vi "CRYTree Refresh Configure Info.vi"(0 "sOption":string, 5 "Step":T1 {"Repeat State Array"."Start" format="%#_5g"; "Y dB ref" format="%.1f"; "Y data" items=["dB", "Lin"]; "Start" format="%#_5g"}, 7 "Item Indent":i32, 9 "Child3":string, 11 "Child4":string, 12 "SpaceStr":string, 13 "Child5":string) -> (4 "Tree Items":T2(array[cluster]))   [LabVIEW 2013]
uses:
  CRYSystem/Typedef Control/CRYStep.ctl
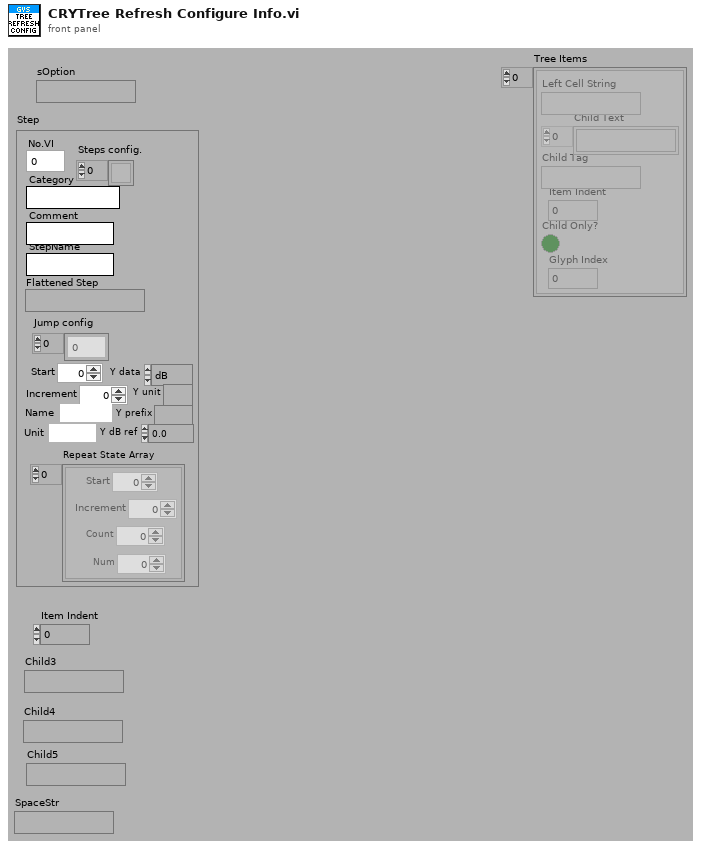
[diagram p1: front panel]
types:
  T1 = typedef "CRYStep.ctl" = cluster{"No.VI":i32, "Category":string, "StepName":string, "Seq setup flattened":string, "Comment":string, "Steps config.":bool[], "Jump config":i32[], "Start":dbl, "Increment":dbl, "Name":string, "Unit":string, "Y data":u16, "Y prefix":string, "Y dB ref":dbl, "Y unit":string, "Repeat State Array":cluster{"Start":dbl, "Increment":dbl, "Count":i32, "Num":i32}[]}
  T2 = cluster{"Left Cell String":string, "Child Text":string[], "Child Tag":string, "Item Indent":i32, "Child Only?":bool, "Glyph Index":i32}[]
  T3 = cluster{"Left Cell String":string, "Child Text":string[], "Child Tag":string, "Item Indent":i32, "Child Only?":bool, "Glyph Index":i32}
  T4 = typedef "CRYStart Cluster.ctl" = cluster{"SequenceName":string, "Preload Stimulus":bool, "CloseOpenedDisplay":bool, "ClearMeasuredData":bool, "UpdateDisplayDuringRun":bool, "DisplayForConfirmation":bool, "HaltOnFail":bool, "UseSameHardware":bool, "UseSameCalibration":bool}
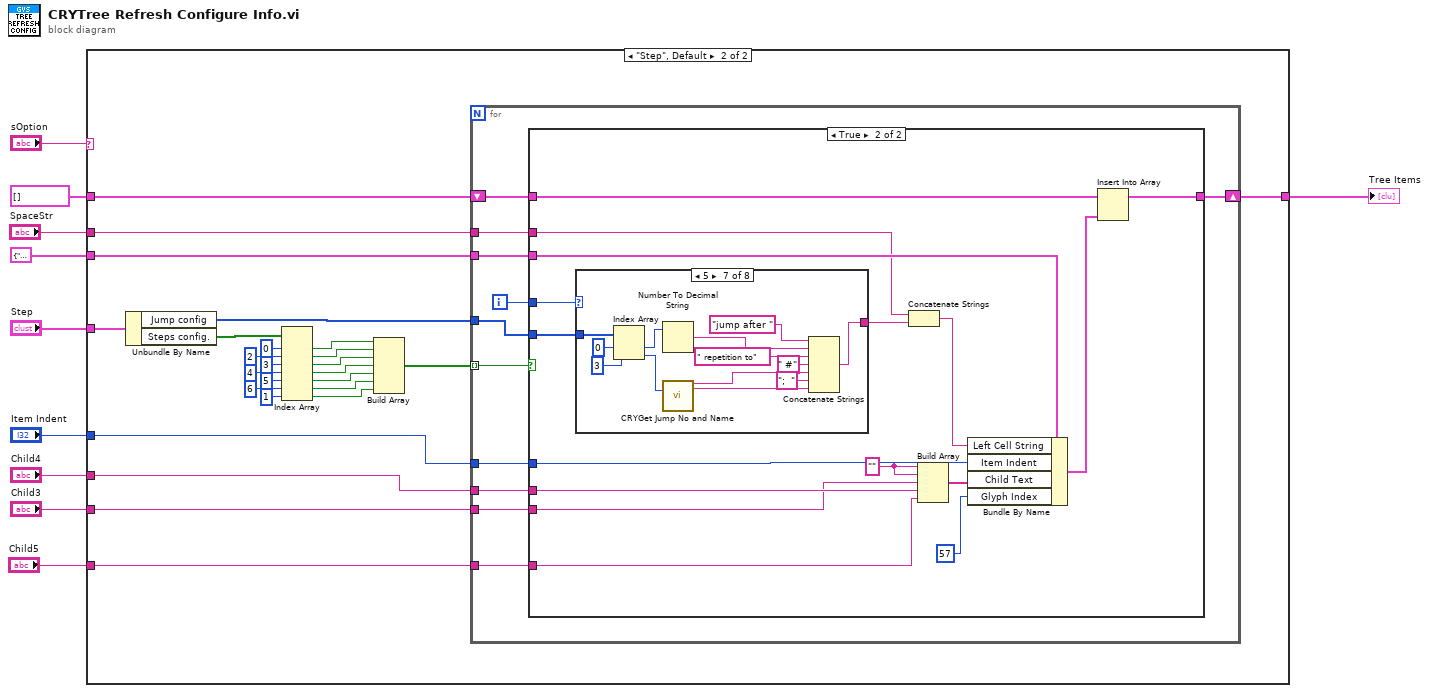
[diagram p0: block diagram]
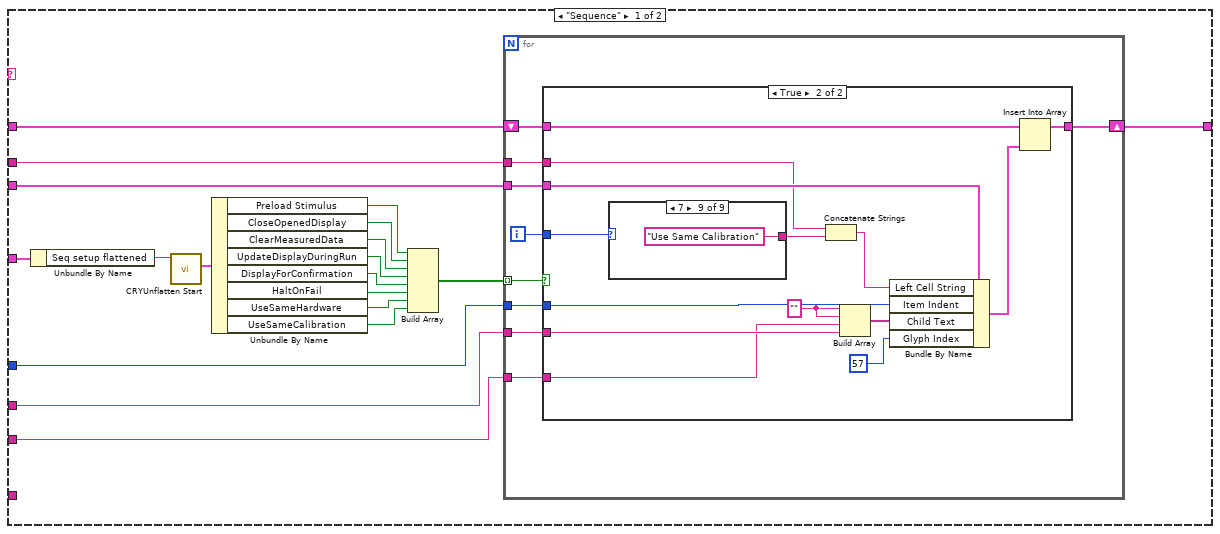
[diagram p2: hidden frame]
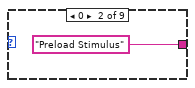
[diagram p5: hidden frame]
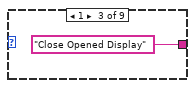
[diagram p6: hidden frame]
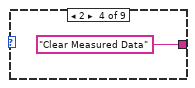
[diagram p7: hidden frame]
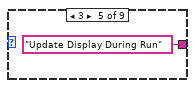
[diagram p8: hidden frame]
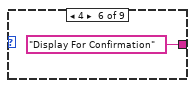
[diagram p9: hidden frame]
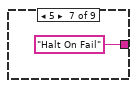
[diagram p10: hidden frame]
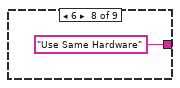
[diagram p11: hidden frame]
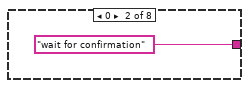
[diagram p14: hidden frame]
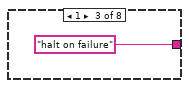
[diagram p15: hidden frame]
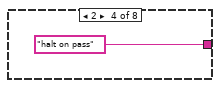
[diagram p16: hidden frame]
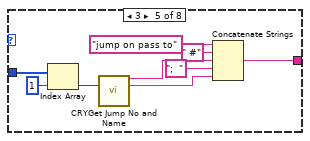
[diagram p17: hidden frame]
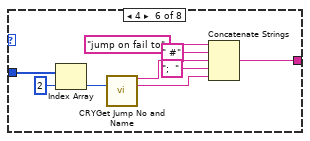
[diagram p18: hidden frame]
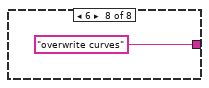
[diagram p19: hidden frame]
diagram:
  n1 = case shown="\"Step\", Default" "sOption" {
    tunnel: T3 {"Left Cell String"="", "Child Text"=[], "Child Tag"="", "Item Indent"=0, "Child Only?"=FALSE, "Glyph Index"=0} ("Item") -> [w24 w84]
    tunnel: T2 [] -> [w23 w83]
    tunnel: [w22 w82] -> w10
    tunnel: "Item Indent" -> [w28 w87]
    tunnel: "Child4" -> [w27 w86]
    tunnel: "Step" -> [w26 w85]
    tunnel: "Child3" -> [w12 w65]
    tunnel: "SpaceStr" -> [w11 w63]
    tunnel: "Child5" -> [_ w62]
    frame "Sequence" {
      n2 = Unbundle By Name(w26) -> ("Seq setup flattened"=w25:string)
      n3 = call "CRYUnflatten Start.vi"("Unflatten Sequence"=w25) -> ("Sequence Configure"=w29:T4)  [unwired: 8 in, 2 out]
      n4 = Unbundle By Name(w29) -> ("Preload Stimulus"=w21:bool, "CloseOpenedDisplay"=w20:bool, "ClearMeasuredData"=w19:bool, "UpdateDisplayDuringRun"=w18:bool, "DisplayForConfirmation"=w17:bool, "HaltOnFail"=w16:bool, "UseSameHardware"=w15:bool, "UseSameCalibration"=w14:bool)
      n5 = Build Array(w21, w20, w19, w18, w17, w16, w15, w14) -> (w13:bool[])
      n6 = for {
        tunnel: w28 -> [w38]
        tunnel: w27 -> [w37]
        tunnel: w24 -> [w36]
        shift-right: [w34] -> w22
        shift-left: w23 -> [w35]
        tunnel: w13 -> [w33] mode=indexing
        tunnel: w12 -> [w31]
        tunnel: w11 -> [w30]
        i -> [w32]
        n7 = case shown="True" w33 {
          tunnel: w38 -> [_ w52]
          tunnel: w37 -> [_ w51]
          tunnel: w36 -> [_ w49]
          tunnel: w35 -> [w39 w48]
          tunnel: [w39 w46] -> w34
          tunnel: w32 -> [_ w45]
          tunnel: w31 -> [_ w41]
          tunnel: w30 -> [_ w40]
          frame False {
          }
          frame True {
            w50 = "" ("SequenceName")
            n8 = case shown="7" w45 {
              tunnel: [_ "Preload Stimulus" ("SequenceName") "Close Opened Display" ("SequenceName") "Clear Measured Data" ("SequenceName") "Update Display During Run" ("SequenceName") "Display For Confirmation" ("SequenceName") "Halt On Fail" ("SequenceName") "Use Same Hardware" ("SequenceName") "Use Same Calibration" ("SequenceName")] -> w43
              frame Default {
              }
              frame 0 {
              }
              frame 1 {
              }
              frame 2 {
              }
              frame 3 {
              }
              frame 4 {
              }
              frame 5 {
              }
              frame 6 {
              }
              frame 7 {
              }
            }
            n9 = Concatenate Strings(w40, w43) -> (w42:string)
            n10 = Build Array(w50, w50, w41, w51) -> (w53:string[])
            n11 = Bundle By Name(cluster=w49, "Left Cell String"=w42, "Item Indent"=w52, "Child Text"=w53, "Glyph Index"=57) -> (w47:T3)
            n12 = Insert Into Array(array=w48, new element=w47) -> (w46:T2)  [unwired: 1 in]
          }
        }
      }
    }
    frame "Step", Default {
      n13 = Unbundle By Name(w85) -> ("Jump config"=w64:i32[], "Steps config."=w80:bool[])
      n14 = Index Array(array=w80, index #1=0 ("index"), index #2=2 ("index"), index #3=3 ("index"), index #4=4 ("index"), index #5=5 ("index"), index #6=6 ("index"), index #7=1 ("index")) -> (element #1=w72:bool, element #2=w71:bool, element #3=w70:bool, element #4=w69:bool, element #5=w68:bool, element #6=w67:bool, element #7=w66:bool)
      n15 = Build Array(w72, w71, w70, w69, w68, w67, w66) -> (w81:bool[])
      n16 = for {
        tunnel: w87 -> [w98]
        tunnel: w86 -> [w97]
        tunnel: w84 -> [w96]
        shift-right: [w94] -> w82
        shift-left: w83 -> [w95]
        tunnel: w81 -> [w93] mode=indexing
        tunnel: w65 -> [w91]
        tunnel: w64 -> [w90]
        tunnel: w63 -> [w89]
        tunnel: w62 -> [w88]
        i -> [w92]
        n17 = case shown="True" w93 {
          tunnel: w98 -> [_ w114]
          tunnel: w97 -> [_ w113]
          tunnel: w96 -> [_ w111]
          tunnel: w95 -> [w99 w110]
          tunnel: [w99 w108] -> w94
          tunnel: w92 -> [_ w107]
          tunnel: w91 -> [_ w103]
          tunnel: w90 -> [_ w102]
          tunnel: w89 -> [_ w101]
          tunnel: w88 -> [_ w100]
          frame False {
          }
          frame True {
            w112 = "" ("SequenceName")
            n18 = case shown="5" w107 {
              tunnel: [_ "wait for confirmation" ("SequenceName") "halt on failure" ("SequenceName") "halt on pass" ("SequenceName") w123 w128 w143 "overwrite curves" ("SequenceName")] -> w105
              tunnel: w102 -> [_ _ _ _ w126 w129 w144 _]
              frame Default {
              }
              frame 0 {
              }
              frame 1 {
              }
              frame 2 {
              }
              frame 3 {
                n19 = Index Array(array=w126, index=1) -> (element=w124:i32)
                n20 = call "CRYGet Jump No and Name.vi"("Jump No"=w124) -> ("Active Cell String1"=w121:string, "Active Cell String0"=w119:string)  [unwired: 13 in]
                n21 = Concatenate Strings("jump on pass to" ("SequenceName"), " #" ("string"), w121, ";  " ("string"), w119) -> (w123:string)
              }
              frame 4 {
                n22 = Index Array(array=w129, index=2) -> (element=w135:i32)
                n23 = call "CRYGet Jump No and Name.vi"("Jump No"=w135) -> ("Active Cell String1"=w133:string, "Active Cell String0"=w131:string)  [unwired: 13 in]
                n24 = Concatenate Strings("jump on fail to" ("SequenceName"), " #" ("string"), w133, ";  " ("string"), w131) -> (w128:string)
              }
              frame 5 {
                n25 = Index Array(array=w144, index #1=0 ("index"), index #2=3 ("index")) -> (element #1=w140:i32, element #2=w141:i32)
                n26 = Number To Decimal String(number=w140) -> (decimal integer string=w139:string)  [unwired: 1 in]
                n27 = call "CRYGet Jump No and Name.vi"("Jump No"=w141) -> ("Active Cell String1"=w147:string, "Active Cell String0"=w145:string)  [unwired: 13 in]
                n28 = Concatenate Strings("jump after " ("SequenceName"), w139, " repetition to" ("string"), " #" ("string"), w147, ";  " ("string"), w145) -> (w143:string)
              }
              frame 6 {
              }
            }
            n29 = Concatenate Strings(w101, w105) -> (w104:string)
            n30 = Build Array(w112, w112, w103, w113, w100) -> (w115:string[])
            n31 = Bundle By Name(cluster=w111, "Left Cell String"=w104, "Item Indent"=w114, "Child Text"=w115, "Glyph Index"=57) -> (w109:T3)
            n32 = Insert Into Array(array=w110, new element=w109) -> (w108:T2)  [unwired: 1 in]
          }
        }
      }
    }
  }
  "Tree Items" <- w10
